vi "UI Language.vi Full Name String.vi"(11 "UI Language.vi Full Name In":string) -> (3 "Actor Core.vi Full Name Out":string)   [LabVIEW 2021]
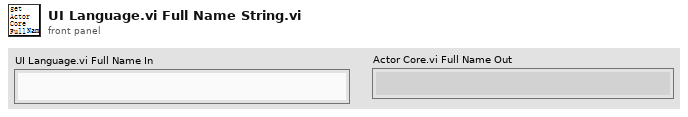
[diagram p1: front panel]
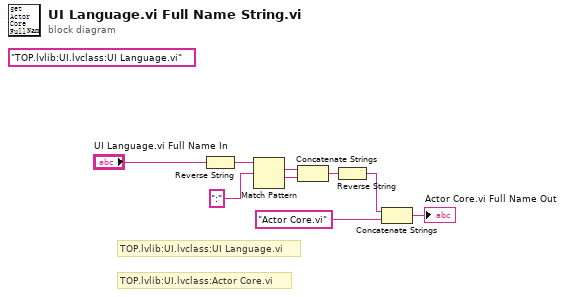
[diagram p0: block diagram]
diagram:
  (unwired) "TOP.lvlib:UI.lvclass:UI Language.vi" ("string")
  # "TOP.lvlib:UI.lvclass:UI Language.vi"
  # "TOP.lvlib:UI.lvclass:Actor Core.vi"
  n1 = Reverse String(1:"UI Language.vi Full Name In") -> (0:w8:string)
  n2 = Match Pattern(string=w8, regular expression=":") -> (match substring=w6:string, after substring=w5:string)  [unwired: 1 in, 2 out]
  n3 = Concatenate Strings(w6, w5) -> (w4:string)
  n4 = Reverse String(1:w4) -> (0:w2:string)
  n5 = Concatenate Strings(w2, "Actor Core.vi" ("reversed")) -> (→"Actor Core.vi Full Name Out":string)
